vi "Create.vi"(8 "error in (no error)":errorcluster) -> (0 "error out":errorcluster, 3 "ConcreteProductA out":refnum<class "ConcreteProductB.lvclass">)   [LabVIEW 2020, in "FactoryMethod.lvlib" / "ConcreteProductB.lvclass"]
uses:
  ConcreteProductB.lvclass
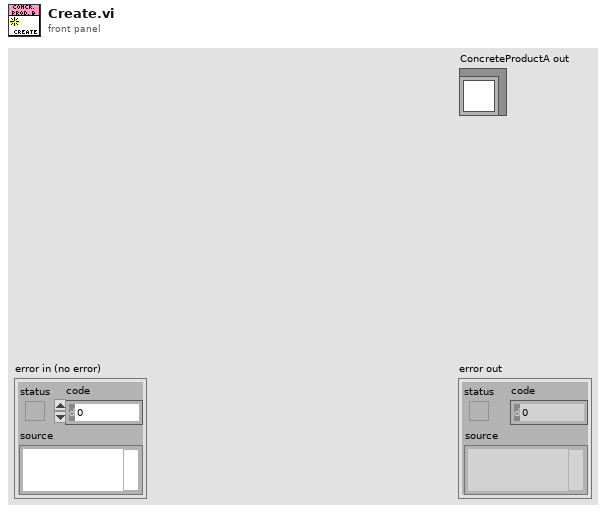
[diagram p1: front panel]
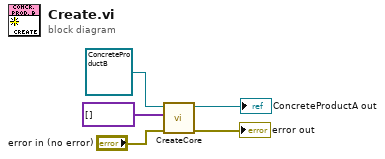
[diagram p0: block diagram]
diagram:
  n1 = call-dynamic "CreateCore.vi"("error in (no error)"="error in (no error)", "ParamsArray"=variant[] [], "ConcreteProductA in"=refnum<class "ConcreteProductB.lvclass"> refnum) -> ("error out"=→"error out":errorcluster, "ConcreteProductA out"=→"ConcreteProductA out":refnum<class "ConcreteProductB.lvclass">)  [unwired: 7 in]
